vi "Debug_Convert_Data_to_String.vi"(8 "error in (no error)":errorcluster, 11 "AB_Source_VI in":refnum<class "AB_Source_VI.lvclass">) -> (0 "error out":errorcluster, 1 "classData":string, 2 "sourceType":string, 3 "AB_Source_VI out":refnum<class "AB_Source_VI.lvclass">)   [LabVIEW 2020, in "AB_Source_VI.lvclass"]
uses:
  <vilib>/AppBuilder/AB_Classes/Source/VI/AB_Source_VI.lvclass
  <vilib>/AppBuilder/AB_Classes/Source/VI/AB_Source_VI.lvclass/AB_Source_VI.ctl
  <vilib>/AppBuilder/AB_Classes/Source/AB_Source.lvclass
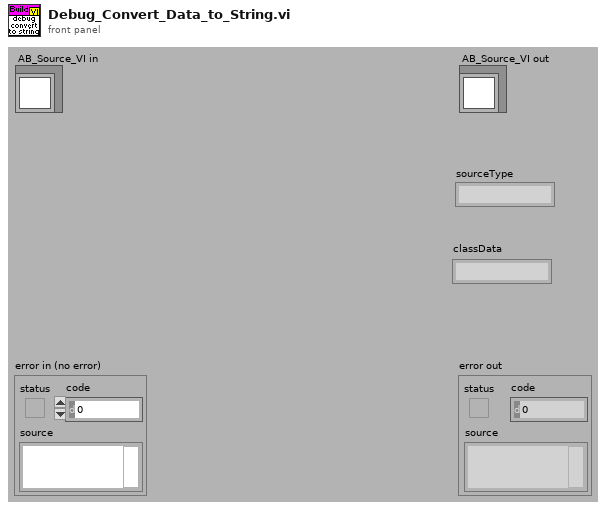
[diagram p1: front panel]
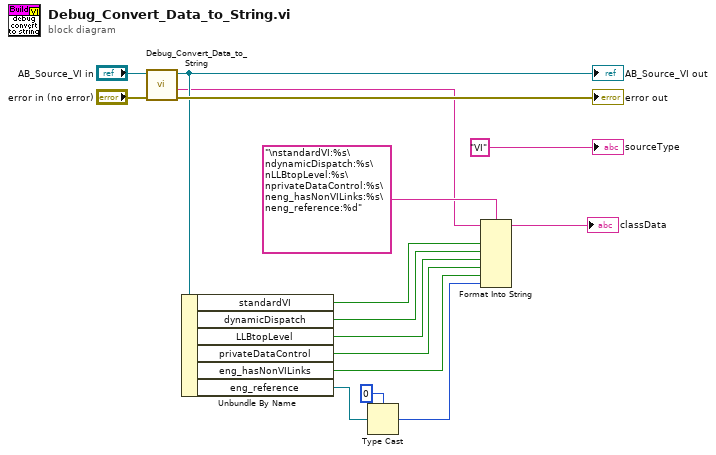
[diagram p0: block diagram]
diagram:
  n1 = call-parent "Debug_Convert_Data_to_String.vi"("error in (no error)"="error in (no error)", "AB_Source in"="AB_Source_VI in") -> ("error out"=→"error out":errorcluster, "classData"=w2:string, "AB_Source out"=w11:refnum<class "AB_Source_VI.lvclass">)  [unwired: 6 in, 1 out]
  "AB_Source_VI out" <- w11
  n2 = Unbundle By Name(w11) -> ("standardVI"=w12:bool, "dynamicDispatch"=w10:bool, "LLBtopLevel"=w9:bool, "privateDataControl"=w1:bool, "eng_hasNonVILinks"=w8:bool, "eng_reference"=w7:refnum<vi>)
  n3 = Type Cast(type=u32 0, x=w7) -> (*(type *) &x=w5:u32)
  n4 = Format Into String(format string="\nstandardVI:%s\ndynamicDispatch:%s\nLLBtopLevel:%s\nprivateDataControl:%s\neng_hasNonVILinks:%s\neng_reference:%d", initial string=w2, w12, w10, w9, w1, w8, w5) -> (resulting string=→"classData":string)  [unwired: 1 in, 1 out]
  "sourceType" <- "VI"
